vi "Set Manual Mode.vi"(6 "Heater Range (0: Off)":u16(ring) items=["Off", "Low (0.5W)", "Med (5W)", "High (50W)"], 7 "Channel (1)":i32=1 min=1 max=4 step=1, 8 "error in (no error)":errorcluster, 9 "Power":dbl, 10 "Manual Mode":bool, 11 "Lakeshore 336 in":refnum<class "Lakeshore 336.lvclass">) -> (0 "error out":errorcluster, 3 "Lakeshore 336 out":refnum<class "Lakeshore 336.lvclass">)   [LabVIEW 2022 SP3, in "Lakeshore 336.lvclass"]
uses:
  Lakeshore 336.lvclass
  Lakeshore 336.lvclass/Lakeshore 336.ctl
  <instrlib>/Lake Shore 336/Lake Shore 336.lvlib
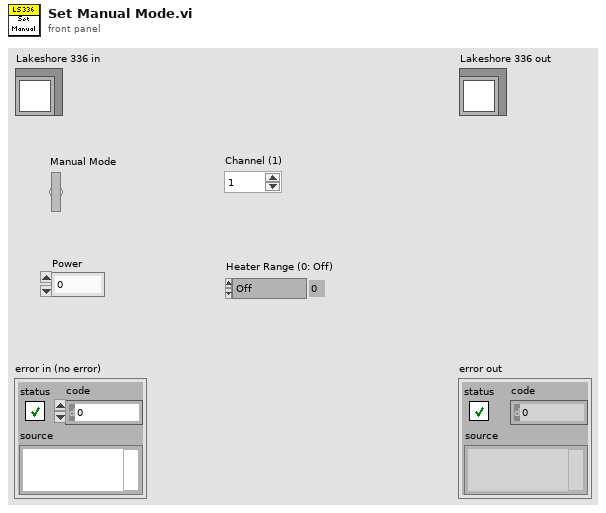
[diagram p1: front panel]
types:
  T1 = typedef "Lakeshore 336.lvclass/Lakeshore 336 Channel Settings cluster.ctl" = cluster{"Input (0:None)":u16, "Power Up Enable (F: Off)":bool, "Mode (0:Off)":u16, "Max Current (0:User Specified)":u16, "Heater Out Display (1:Current)":u16, "Max User Current (2.000)":dbl, "Heater Resistance (1:25 Ohms)":u16, "PID":T2, "Name":string}
  T2 = typedef "Lakeshore 336.lvclass/Lakeshore 336 PID cluster.ctl" = cluster{"P":dbl, "I":dbl, "D":dbl}
  T3 = typedef "Lakeshore 336.lvclass/Lakeshore 336 Settings cluster.ctl" = cluster{"Lake Shore 336 Address":refnum<visa-resource-name>, "Output Ch":T1[], "Input Ch":T4[], "Prefix":string, "Setpoints":dbl[]}
  T4 = typedef "Lakeshore 336.lvclass/Lakeshore 336 Input Ch config cluster.ctl" = cluster{"Name":string}
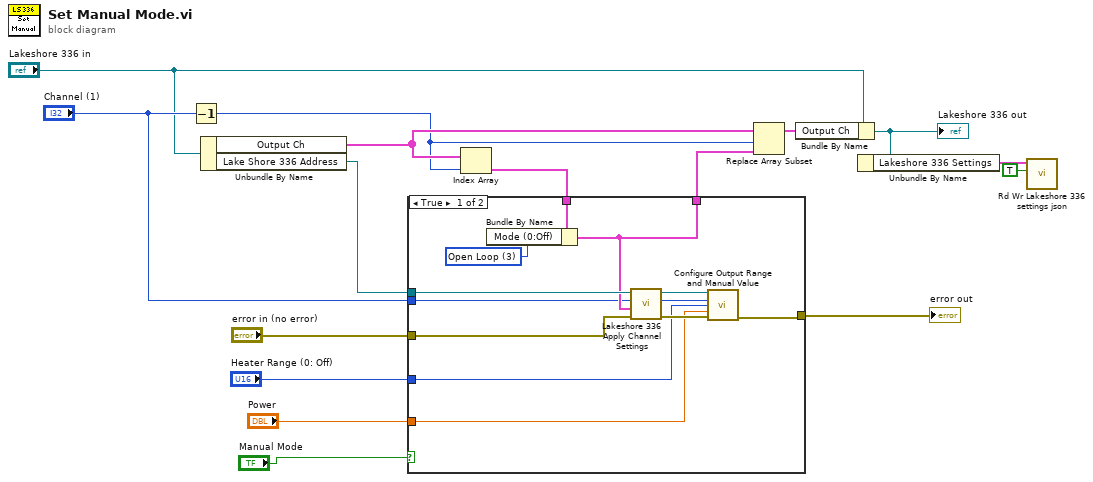
[diagram p0: block diagram]
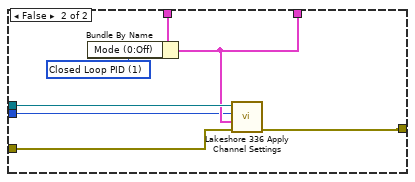
[diagram p2: hidden frame]
diagram:
  n1 = Decrement(x="Channel (1)") -> (x-1=w13:i32)
  n2 = Unbundle By Name("Lakeshore 336 in") -> ("Output Ch"=w14:T1[], "Lake Shore 336 Address"=w15:refnum<visa-resource-name>)
  n3 = Index Array(array=w14, index=w13) -> (element=w16:T1)
  n4 = case shown="True" "Manual Mode" {
    tunnel: w16 -> [w28 w35]
    tunnel: w15 -> [w26 w33]
    tunnel: [w25 w32] -> w12
    tunnel: "Channel (1)" -> [w22 w31]
    tunnel: "error in (no error)" -> [w20 w30]
    tunnel: "Power" -> [w19 _]
    tunnel: "Heater Range (0: Off)" -> [w18 _]
    tunnel: [w17 w29] -> w4
    frame True {
      w27 = u16 3 items=["Off", "Closed Loop PID", "Zone", "Open Loop"] ("Mode (0:Off)")
      n5 = Bundle By Name(cluster=w28, "Mode (0:Off)"=w27) -> (w25:T1)
      n6 = call "Lakeshore 336 Apply Channel Settings.vi"("error in (no error)"=w20, "Manual Settings"=w25, "Channel (1)"=w22, "Addr"=w26) -> ("error out"=w23:errorcluster, "Channel dup"=w21:i32, "Addr dup"=w24:refnum<visa-resource-name>)  [unwired: 5 in]
      n7 = call <instrlib>:"Configure Output Range and Manual Value.vi"("VISA resource name"=w24, "Output (1:1)"=w21, "Range (0:Off)"=w18, "Manual Output (0.00 %)"=w19, "error in (no error)"=w23) -> ("error out"=w17:errorcluster)  [unwired: 9 in, 1 out]
    }
    frame False {
      w34 = u16 1 items=["Off", "Closed Loop PID", "Zone", "Open Loop"] ("Mode (0:Off)")
      n8 = Bundle By Name(cluster=w35, "Mode (0:Off)"=w34) -> (w32:T1)
      n9 = call "Lakeshore 336 Apply Channel Settings.vi"("error in (no error)"=w30, "Manual Settings"=w32, "Channel (1)"=w31, "Addr"=w33) -> ("error out"=w29:errorcluster)  [unwired: 5 in, 2 out]
    }
  }
  "error out" <- w4
  n10 = Replace Array Subset(array=w14, new element=w12, index=w13) -> (w11:T1[])
  n11 = Bundle By Name(cluster="Lakeshore 336 in", "Output Ch"=w11) -> (w3:refnum<class "Lakeshore 336.lvclass">)
  "Lakeshore 336 out" <- w3
  n12 = Unbundle By Name(w3) -> ("Lakeshore 336 Settings"=w2:T3)
  n13 = call "Rd Wr Lakeshore 336 settings json.vi"("Write? (F:Read)"=TRUE, "Lakeshore 336 Settings"=w2) -> ()  [unwired: 8 in, 2 out]
